vi "end cube--C1.vi"(7 "Switch":string, 8 "Command Info In":T1, 10 "end cube--C1":T5, 11 "Starting Position":T4) -> (0 "Command Info Out":T1)   [LabVIEW 2017]
uses:
  Block Clusters/end cube--C1.ctl
  <vilib>/Rock Robotics/WPI/Framework/Command Status Info.ctl
  <vilib>/Rock Robotics/WPI/Framework/Completion Status.ctl
  <vilib>/Rock Robotics/WPI/Framework/Completion Notifier.ctl
  Support Code/Starting Position.ctl
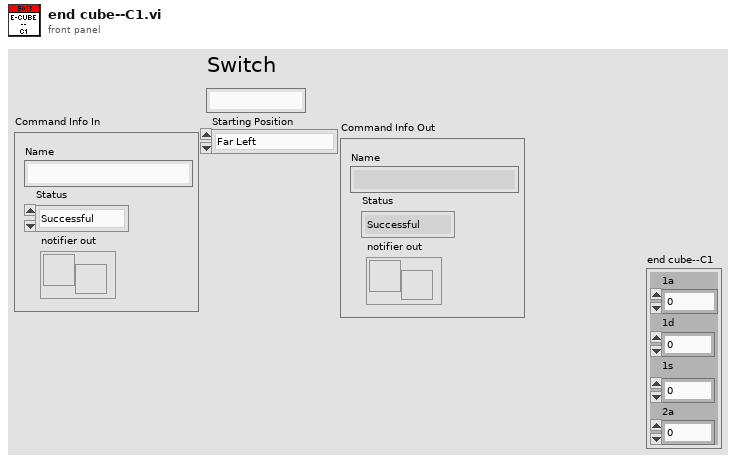
[diagram p1: front panel]
types:
  T1 = typedef "Command Status Info.ctl" = cluster{"Name":string, "Status":T2, "notifier out":T3}
  T2 = typedef "Completion Status.ctl" = enum16{"Successful", "Aborted", "Incomplete"}
  T3 = typedef "Completion Notifier.ctl" = refnum<notifier>
  T4 = typedef "Starting Position.ctl" = enum16{"Far Left", "Middle", "Far Right"}
  T5 = typedef "end cube--C1.ctl" = cluster{"1a":dbl, "1d":dbl, "1s":dbl, "2a":dbl}
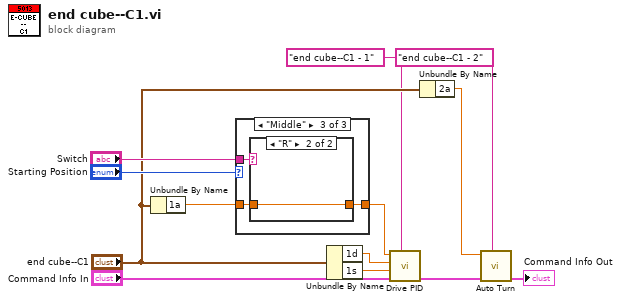
[diagram p0: block diagram]
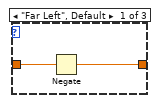
[diagram p2: hidden frame]
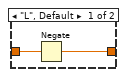
[diagram p4: hidden frame]
diagram:
  n1 = Unbundle By Name("end cube--C1") -> ("1a"=w6:dbl)
  n2 = case shown="\"Middle\"" "Starting Position" {
    tunnel: w6 -> [w15 w16 w19]
    tunnel: [w14 w16 w17] -> w10
    tunnel: "Switch" -> [_ _ w18]
    frame "Far Left", Default {
      n3 = Negate(x=w15) -> (-x=w14:dbl)
    }
    frame "Far Right" {
    }
    frame "Middle" {
      n4 = case shown="\"R\"" w18 {
        tunnel: [w21 w22] -> w17
        tunnel: w19 -> [w20 w22]
        frame "L", Default {
          n5 = Negate(x=w20) -> (-x=w21:dbl)
        }
        frame "R" {
        }
      }
    }
  }
  n6 = Unbundle By Name("end cube--C1") -> ("1d"=w7:dbl, "1s"=w8:dbl)
  n7 = call "Drive PID.vi"("Description"="end cube--C1 - 1", "Command Info In"="Command Info In", "Speed"=w8, "Distance"=w7, "Target Angle"=w10) -> ("Command Info Out"=w13:T1)  [unwired: 6 in]
  n8 = Unbundle By Name("end cube--C1") -> ("2a"=w3:dbl)
  n9 = call "Auto Turn.vi"("Description"="end cube--C1 - 2", "Command Info In"=w13, "Target Angle"=w3) -> ("Command Info Out"=→"Command Info Out":T1)  [unwired: 8 in]
